vi "VI Anlagengrenzwerte Amium PNS.vi"() -> ()   [LabVIEW 2020, in "Amium PNS.lvlib"]
uses:
  Amium PNS/Amium PNS.lvlib
  Amium PNS/Amium Anlagengrenzwerte PNS.ctl
  Amium PNS/Amium Anlagengrenzwerte-Parameter Anzeige.ctl
  Visualisierungs Elemente/Zahlen-Eingabefeld.ctl
  Visualisierungs Elemente/Button.ctl
  Visualisierungs Elemente/Zahlen-Ausgabefeld.ctl
  Amium PNS/PNS Istwerte_Amium.ctl
  Amium PNS/Amium ErrorCluster.ctl
  Amium PNS/Amium Zustand.ctl
  Amium PNS/SP_Daten.ctl
  Amium PNS/Aktion FGV Amium Daten.ctl
  Seiten/System Einstellungen V2/Aktioen FGV System.ctl
  Amium PNS/AK Kommunikation/Amium Kommandos verwalten Aktionen.ctl
  PNS/Diagnose PNS.vi
  Allgemein/allgemeine Sub-VIs.lvlib
  PNS/PNS.lvlib
  PNS/PNS Anlagenuebersicht einfaerben Aktionen.ctl
  Amium PNS/AK Kommunikation/AK Kommunikation.lvlib
  Seiten/System Einstellungen V2/System Einstellungen V2.lvlib
panel:
  in  "SP":T1
  out "Messgasdruck:":sgl format="%#_5g"
  out "Amium Zustände":T2 items=["Pause", "Aufheizphase", "Standby", "Messen", "Spülen", "Leakcheck"]
  out "Entnahmestelle:":sgl[](array[numeric]) format="%#_5g"
  in  "Port:":u32
  out "Software Version:":string
  out "PNS Istwerte":T3 {"Istwert 14" format="%.1f"; "Istwert 13" format="%.1f"; "Istwert 12" format="%.1f"; "Istwert 11" format="%.1f"; "Istwert 10" format="%.1f"; "Istwert 9" format="%.1f"; "Istwert 8" format="%.1f"; "Istwert 7" format="%.1f"; "Istwert 6" format="%.1f"; "Istwert 5" format="%.1f"; "Istwert 4" format="%.1f"; "Istwert 3" format="%.1f"; "Istwert 2" format="%.1f"; "Istwert 1" format="%.1f"}
  in  "IP-Adresse PNS:":string
  out "Seriennummer:":string
  out "Detail Status:":T4 format="%#_5g"
  out "Status:":T4 format="%#_5g"
  out "Druckluft Störung:":T4 format="%#_5g"
  out "AWC IST:":T4 format="%#_5g"
  out "Error Out":errorcluster caption="Fehlercluster"
  in  "Diag PNS":T5
  in  "Grenzwerte PNS":T6={"Filter:"={"Sollwert"=0.0, "Warn-Min"=0.0, "Warn-Max"=0.0, "Abschalt-Min"=0.0, "Abschalt-Max"=0.0, "Regler"=1}, "Ventilplatte:"={"Sollwert"=0.0, "Warn-Min"=0.0, "Warn-Max"=0.0, "Abschalt-Min"=0.0, "Abschalt-Max"=0.0, "Regler"=1}, "Heizleitung 1:"={"Sollwert"=0.0, "Warn-Min"=0.0, "Warn-Max"=0.0, "Abschalt-Min"=0.0, "Abschalt-Max"=0.0, "Regler"=1}, "Heizleitung 2:"={"Sollwert"=0.0, "Warn-Min"=0.0, "Warn-Max"=0.0, "Abschalt-Min"=0.0, "Abschalt-Max"=0.0, "Regler"=1}, "Heizleitung 3:"={"Sollwert"=0.0, "Warn-Min"=0.0, "Warn-Max"=0.0, "Abschalt-Min"=0.0, "Abschalt-Max"=0.0, "Regler"=1}, "Heizleitung 4:"={"Sollwert"=0.0, "Warn-Min"=0.0, "Warn-Max"=0.0, "Abschalt-Min"=0.0, "Abschalt-Max"=0.0, "Regler"=1}, "Heizleitung 5:"={"Sollwert"=0.0, "Warn-Min"=0.0, "Warn-Max"=0.0, "Abschalt-Min"=0.0, "Abschalt-Max"=0.0, "Regler"=1}, "Heizleitung 6:"={"Sollwert"=0.0, "Warn-Min"=0.0, "Warn-Max"=0.0, "Abschalt-Min"=0.0, "Abschalt-Max"=0.0, "Regler"=1}, "Heizleitung 7:"={"Sollwert"=0.0, "Warn-Min"=0.0, "Warn-Max"=0.0, "Abschalt-Min"=0.0, "Abschalt-Max"=1.0, "Regler"=1}, "Heizleitung 8:"={"Sollwert"=0.0, "Warn-Min"=0.0, "Warn-Max"=0.0, "Abschalt-Min"=0.0, "Abschalt-Max"=0.0, "Regler"=1}, "Heizleitung 9:"={"Sollwert"=0.0, "Warn-Min"=0.0, "Warn-Max"=0.0, "Abschalt-Min"=0.0, "Abschalt-Max"=0.0, "Regler"=1}, "Heizleitung 10:"={"Sollwert"=0.0, "Warn-Min"=0.0, "Warn-Max"=0.0, "Abschalt-Min"=0.0, "Abschalt-Max"=0.0, "Regler"=1}, "Heizleitung 11:"={"Sollwert"=0.0, "Warn-Min"=0.0, "Warn-Max"=0.0, "Abschalt-Min"=0.0, "Abschalt-Max"=0.0, "Regler"=1}, "Heizleitung 12:"={"Sollwert"=0.0, "Warn-Min"=0.0, "Warn-Max"=0.0, "Abschalt-Min"=0.0, "Abschalt-Max"=0.0, "Regler"=1}} {"Heizleitung 12:"."Regler" items=["aktiv", "inaktiv"]; "Heizleitung 12:"."Abschalt-Max" format="%#_5g"; "Heizleitung 12:"."Abschalt-Min" format="%#_5g"; "Heizleitung 12:"."Warn-Max" format="%#_5g"; "Heizleitung 12:"."Warn-Min" format="%#_5g"; "Heizleitung 12:"."Sollwert" format="%#_5g"; "Heizleitung 11:"."Regler" items=["aktiv", "inaktiv"]; "Heizleitung 11:"."Abschalt-Max" format="%#_5g"; "Heizleitung 11:"."Abschalt-Min" format="%#_5g"; "Heizleitung 11:"."Warn-Max" format="%#_5g"; "Heizleitung 11:"."Warn-Min" format="%#_5g"; "Heizleitung 11:"."Sollwert" format="%#_5g"; "Heizleitung 10:"."Regler" items=["aktiv", "inaktiv"]; "Heizleitung 10:"."Abschalt-Max" format="%#_5g"; "Heizleitung 10:"."Abschalt-Min" format="%#_5g"; "Heizleitung 10:"."Warn-Max" format="%#_5g"; "Heizleitung 10:"."Warn-Min" format="%#_5g"; "Heizleitung 10:"."Sollwert" format="%#_5g"; "Heizleitung 9:"."Regler" items=["aktiv", "inaktiv"]; "Heizleitung 9:"."Abschalt-Max" format="%#_5g"; "Heizleitung 9:"."Abschalt-Min" format="%#_5g"; "Heizleitung 9:"."Warn-Max" format="%#_5g"; "Heizleitung 9:"."Warn-Min" format="%#_5g"; "Heizleitung 9:"."Sollwert" format="%#_5g"; "Heizleitung 8:"."Regler" items=["aktiv", "inaktiv"]; "Heizleitung 8:"."Abschalt-Max" format="%#_5g"; "Heizleitung 8:"."Abschalt-Min" format="%#_5g"; "Heizleitung 8:"."Warn-Max" format="%#_5g"; "Heizleitung 8:"."Warn-Min" format="%#_5g"; "Heizleitung 8:"."Sollwert" format="%#_5g"; "Heizleitung 7:"."Regler" items=["aktiv", "inaktiv"]; "Heizleitung 7:"."Abschalt-Max" format="%#_5g"; "Heizleitung 7:"."Abschalt-Min" format="%#_5g"; "Heizleitung 7:"."Warn-Max" format="%#_5g"; "Heizleitung 7:"."Warn-Min" format="%#_5g"; "Heizleitung 7:"."Sollwert" format="%#_5g"; "Heizleitung 6:"."Regler" items=["aktiv", "inaktiv"]; "Heizleitung 6:"."Abschalt-Max" format="%#_5g"; "Heizleitung 6:"."Abschalt-Min" format="%#_5g"; "Heizleitung 6:"."Warn-Max" format="%#_5g"; "Heizleitung 6:"."Warn-Min" format="%#_5g"; "Heizleitung 6:"."Sollwert" format="%#_5g"; "Heizleitung 5:"."Regler" items=["aktiv", "inaktiv"]; "Heizleitung 5:"."Abschalt-Max" format="%#_5g"; "Heizleitung 5:"."Abschalt-Min" format="%#_5g"; "Heizleitung 5:"."Warn-Max" format="%#_5g"; "Heizleitung 5:"."Warn-Min" format="%#_5g"; "Heizleitung 5:"."Sollwert" format="%#_5g"; "Heizleitung 4:"."Regler" items=["aktiv", "inaktiv"]; "Heizleitung 4:"."Abschalt-Max" format="%#_5g"; "Heizleitung 4:"."Abschalt-Min" format="%#_5g"; "Heizleitung 4:"."Warn-Max" format="%#_5g"; "Heizleitung 4:"."Warn-Min" format="%#_5g"; "Heizleitung 4:"."Sollwert" format="%#_5g"; "Heizleitung 3:"."Regler" items=["aktiv", "inaktiv"]; "Heizleitung 3:"."Abschalt-Max" format="%#_5g"; "Heizleitung 3:"."Abschalt-Min" format="%#_5g"; "Heizleitung 3:"."Warn-Max" format="%#_5g"; "Heizleitung 3:"."Warn-Min" format="%#_5g"; "Heizleitung 3:"."Sollwert" format="%#_5g"; "Heizleitung 2:"."Regler" items=["aktiv", "inaktiv"]; "Heizleitung 2:"."Abschalt-Max" format="%#_5g"; "Heizleitung 2:"."Abschalt-Min" format="%#_5g"; "Heizleitung 2:"."Warn-Max" format="%#_5g"; "Heizleitung 2:"."Warn-Min" format="%#_5g"; "Heizleitung 2:"."Sollwert" format="%#_5g"; "Heizleitung 1:"."Regler" items=["aktiv", "inaktiv"]; "Heizleitung 1:"."Abschalt-Max" format="%#_5g"; "Heizleitung 1:"."Abschalt-Min" format="%#_5g"; "Heizleitung 1:"."Warn-Max" format="%#_5g"; "Heizleitung 1:"."Warn-Min" format="%#_5g"; "Heizleitung 1:"."Sollwert" format="%#_5g"; "Ventilplatte:"."Regler" items=["aktiv", "inaktiv"]; "Ventilplatte:"."Abschalt-Max" format="%#_5g"; "Ventilplatte:"."Abschalt-Min" format="%#_5g"; "Ventilplatte:"."Warn-Max" format="%#_5g"; "Ventilplatte:"."Warn-Min" format="%#_5g"; "Ventilplatte:"."Sollwert" format="%#_5g"; "Filter:"."Regler" items=["aktiv", "inaktiv"]; "Filter:"."Abschalt-Max" format="%#_5g"; "Filter:"."Abschalt-Min" format="%#_5g"; "Filter:"."Warn-Max" format="%#_5g"; "Filter:"."Warn-Min" format="%#_5g"; "Filter:"."Sollwert" format="%#_5g"}
  out "Fehler Cluster":T9
  # "Amium Anlagengrenzwerte PNS"
  # "Allgemeine Werte"
  # "Abschaltgrenzen"
  # "Warngrenzen"
  # "Regelung \naktiv/inaktiv"
  # "Parameter"
  # "Istwert"
  # "Sollwert"
  # "Min"
  # "Max"
  # "Min"
  # "Max"
  # "Heizleitung 1:"
  # "Diagnosewerte"
  # "Heizleitung 2:"
  # "Heizleitung 3:"
  # "Heizleitung 4:"
  # "Heizleitung 5:"
  # "Heizleitung 6:"
  # "Heizleitung 7:"
  # "Heizleitung 8:"
  # "Heizleitung 9:"
  # "Heizleitung 10:"
  # "Ofen / Filter:"
  # "HL Zuleitung:"
  # "Wanddurchführung:"
  # "AddOn:"
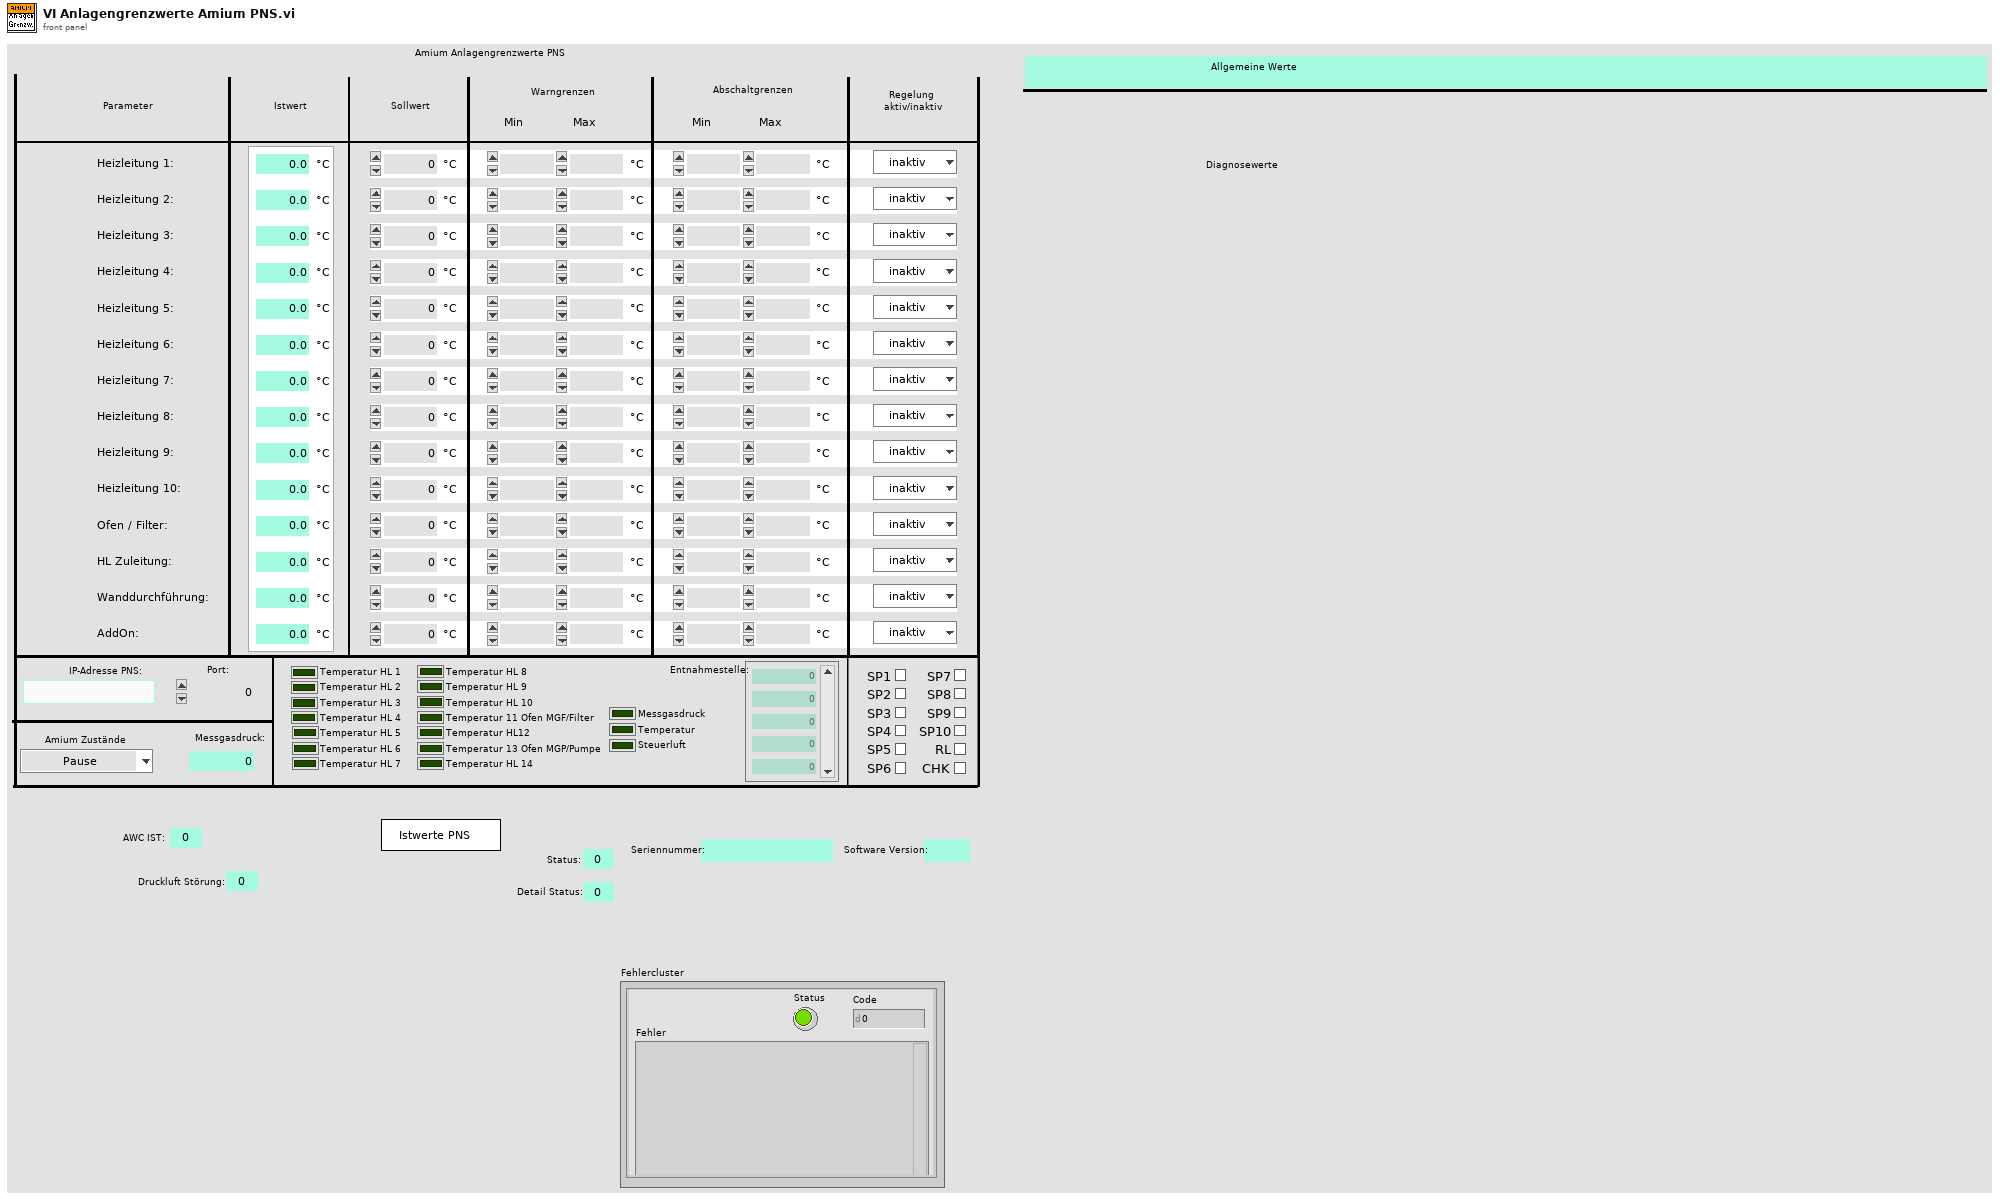
[diagram p1: front panel]
types:
  T1 = typedef "Amium PNS.lvlib/SP_Daten.ctl" = cluster{"SP1":bool, "SP2":bool, "SP3":bool, "SP4":bool, "SP5":bool, "SP6":bool, "SP7":bool, "SP8":bool, "SP9":bool, "SP10":bool, "RL":bool, "CHK":bool}
  T2 = typedef "Amium PNS.lvlib/Amium Zustand.ctl" = u16
  T3 = typedef "Amium PNS.lvlib/PNS Istwerte_Amium.ctl" = cluster{"Istwert 1":sgl, "Istwert 2":sgl, "Istwert 3":sgl, "Istwert 4":sgl, "Istwert 5":sgl, "Istwert 6":sgl, "Istwert 7":sgl, "Istwert 8":sgl, "Istwert 9":sgl, "Istwert 10":sgl, "Istwert 11":sgl, "Istwert 12":sgl, "Istwert 13":sgl, "Istwert 14":sgl}
  T4 = typedef "Zahlen-Ausgabefeld.ctl" = sgl
  T5 = typedef "Button.ctl" = bool
  T6 = typedef "Amium PNS.lvlib/Amium Anlagengrenzwerte PNS.ctl" = cluster{"Filter:":T7, "Ventilplatte:":T7, "Heizleitung 1:":T7, "Heizleitung 2:":T7, "Heizleitung 3:":T7, "Heizleitung 4:":T7, "Heizleitung 5:":T7, "Heizleitung 6:":T7, "Heizleitung 7:":T7, "Heizleitung 8:":T7, "Heizleitung 9:":T7, "Heizleitung 10:":T7, "Heizleitung 11:":T7, "Heizleitung 12:":T7}
  T7 = typedef "Amium PNS.lvlib/Amium Anlagengrenzwerte-Parameter Anzeige.ctl" = cluster{"Sollwert":T8, "Warn-Min":T8, "Warn-Max":T8, "Abschalt-Min":T8, "Abschalt-Max":T8, "Regler":u16}
  T8 = typedef "Zahlen-Eingabefeld.ctl" = sgl
  T9 = typedef "Amium PNS.lvlib/Amium ErrorCluster.ctl" = cluster{"Messgasdruck":bool, "Temperatur":bool, "Steuerluft":bool, "Temperatur HL 1":bool, "Temperatur HL 2":bool, "Temperatur HL 3":bool, "Temperatur HL 4":bool, "Temperatur HL 5":bool, "Temperatur HL 6":bool, "Temperatur HL 7":bool, "Temperatur HL 8":bool, "Temperatur HL 9":bool, "Temperatur HL 10":bool, "Temperatur 11 Ofen MGF/Filter":bool, "Temperatur HL12":bool, "Temperatur 13 Ofen MGP/Pumpe":bool, "Temperatur HL 14":bool}
  T10 = enum8{"Enabled", "Disabled", "Disabled and Grayed Out"}
  T11 = typedef "System Einstellungen V2.lvlib/Aktioen FGV System.ctl" = enum16{"lesen", "laden", "speichern", "Optionen schreiben", "Zeitstempel", "Reset BMP", "Reset SQP", "Wartung", "Werkseinstellung"}
  T12 = typedef "Amium PNS.lvlib/Aktion FGV Amium Daten.ctl" = enum16{"lesen", "Komm Daten", "Daten", "Error", "Regler", "Grenzwerte", "laden", "speichern"}
  T13 = typedef "PNS.lvlib/PNS Anlagenuebersicht einfaerben Aktionen.ctl" = enum16{"lesen", "prüfen", "initialisieren"}
  T14 = typedef "System Einstellungen V2.lvlib/Optionen.ctl" = cluster{"Störmeldep.":bool, "Betriebszustände":bool, "LN2 Befüllung":bool, "Klimaanlage ?":bool, "AK in ppm":bool, "log Cal-Gas":bool, "log 0-Gas":bool, "log CG zu PNS":bool, "Reserve":bool, "Durchflusssensor 0-5V":bool, "PNS?":bool, "Container":bool, "Mit N2 spülen":bool, "Span Gas Auswahl":T15, "VFS 1":bool, "VFS 2":bool, "VFS 3":bool, "VFS 4":bool, "TRE08":bool, "Leakcheck vor Kal":bool, "Amium 10-Fach":bool, "Verticale Scrollbar aktiv":bool, "Loggingtakt":bool, "SP laden speichern":u16}
  T15 = typedef "Funktionstasten.lvlib/Spaneingang.ctl" = u16
  T16 = typedef "Amium PNS.lvlib/Kommunikation Daten Cluster.ctl" = cluster{"IP Adresse":string, "Port":i16}
  T17 = typedef "Amium PNS.lvlib/AK Kommunikation.lvlib/Amium Kommandos verwalten Aktionen.ctl" = enum16{"lesen", "setzen Ende", "setzen Pos1", "senden", "initalisieren", "prüfen", "Kommandos"}
  T18 = cluster{"Filter:":cluster{"Sollwert":bool, "Warn-Min":bool, "Warn-Max":bool, "Abschalt-Min":bool, "Abschalt-Max":bool, "Regler":bool}, "Ventilplatte:":cluster{"Sollwert":bool, "Warn-Min":bool, "Warn-Max":bool, "Abschalt-Min":bool, "Abschalt-Max":bool, "Regler":bool}, "Heizleitung 1:":cluster{"Sollwert":bool, "Warn-Min":bool, "Warn-Max":bool, "Abschalt-Min":bool, "Abschalt-Max":bool, "Regler":bool}, "Heizleitung 2:":cluster{"Sollwert":bool, "Warn-Min":bool, "Warn-Max":bool, "Abschalt-Min":bool, "Abschalt-Max":bool, "Regler":bool}, "Heizleitung 3:":cluster{"Sollwert":bool, "Warn-Min":bool, "Warn-Max":bool, "Abschalt-Min":bool, "Abschalt-Max":bool, "Regler":bool}, "Heizleitung 4:":cluster{"Sollwert":bool, "Warn-Min":bool, "Warn-Max":bool, "Abschalt-Min":bool, "Abschalt-Max":bool, "Regler":bool}, "Heizleitung 5:":cluster{"Sollwert":bool, "Warn-Min":bool, "Warn-Max":bool, "Abschalt-Min":bool, "Abschalt-Max":bool, "Regler":bool}, "Heizleitung 6:":cluster{"Sollwert":bool, "Warn-Min":bool, "Warn-Max":bool, "Abschalt-Min":bool, "Abschalt-Max":bool, "Regler":bool}, "Heizleitung 7:":cluster{"Sollwert":bool, "Warn-Min":bool, "Warn-Max":bool, "Abschalt-Min":bool, "Abschalt-Max":bool, "Regler":bool}, "Heizleitung 8:":cluster{"Sollwert":bool, "Warn-Min":bool, "Warn-Max":bool, "Abschalt-Min":bool, "Abschalt-Max":bool, "Regler":bool}, "Heizleitung 9:":cluster{"Sollwert":bool, "Warn-Min":bool, "Warn-Max":bool, "Abschalt-Min":bool, "Abschalt-Max":bool, "Regler":bool}, "Heizleitung 10:":cluster{"Sollwert":bool, "Warn-Min":bool, "Warn-Max":bool, "Abschalt-Min":bool, "Abschalt-Max":bool, "Regler":bool}, "Heizleitung 11:":cluster{"Sollwert":bool, "Warn-Min":bool, "Warn-Max":bool, "Abschalt-Min":bool, "Abschalt-Max":bool, "Regler":bool}, "Heizleitung 12:":cluster{"Sollwert":bool, "Warn-Min":bool, "Warn-Max":bool, "Abschalt-Min":bool, "Abschalt-Max":bool, "Regler":bool}}
  T19 = cluster{"Sollwert":bool, "Warn-Min":bool, "Warn-Max":bool, "Abschalt-Min":bool, "Abschalt-Max":bool, "Regler":bool}[]
  T20 = typedef "Amium PNS.lvlib/Daten Cluster.ctl" = cluster{"Amium Zustände":T2, "Samplepoint am PNS":i16, "Gerätekennung":string, "aktiver Samplepoint":i16[], "Messgasdruck":sgl}
  T21 = typedef "Amium PNS.lvlib/Temperaturregler Cluster.ctl" = cluster{"Istwert":sgl, "Sollwert":sgl, "Stellgröße":sgl, "Status":sgl, "Error":sgl}
  T22 = cluster{"Istwert":sgl, "Istwert":sgl, "Istwert":sgl, "Istwert":sgl, "Istwert":sgl, "Istwert":sgl, "Istwert":sgl, "Istwert":sgl, "Istwert":sgl, "Istwert":sgl, "Istwert":sgl, "Istwert":sgl, "Istwert":sgl, "Istwert":sgl}
  T23 = cluster{"[0]":T7, "[1]":T7, "[2]":T7, "[3]":T7, "[4]":T7, "[5]":T7, "[6]":T7, "[7]":T7, "[8]":T7, "[9]":T7, "[10]":T7, "[11]":T7, "[12]":T7, "[13]":T7}
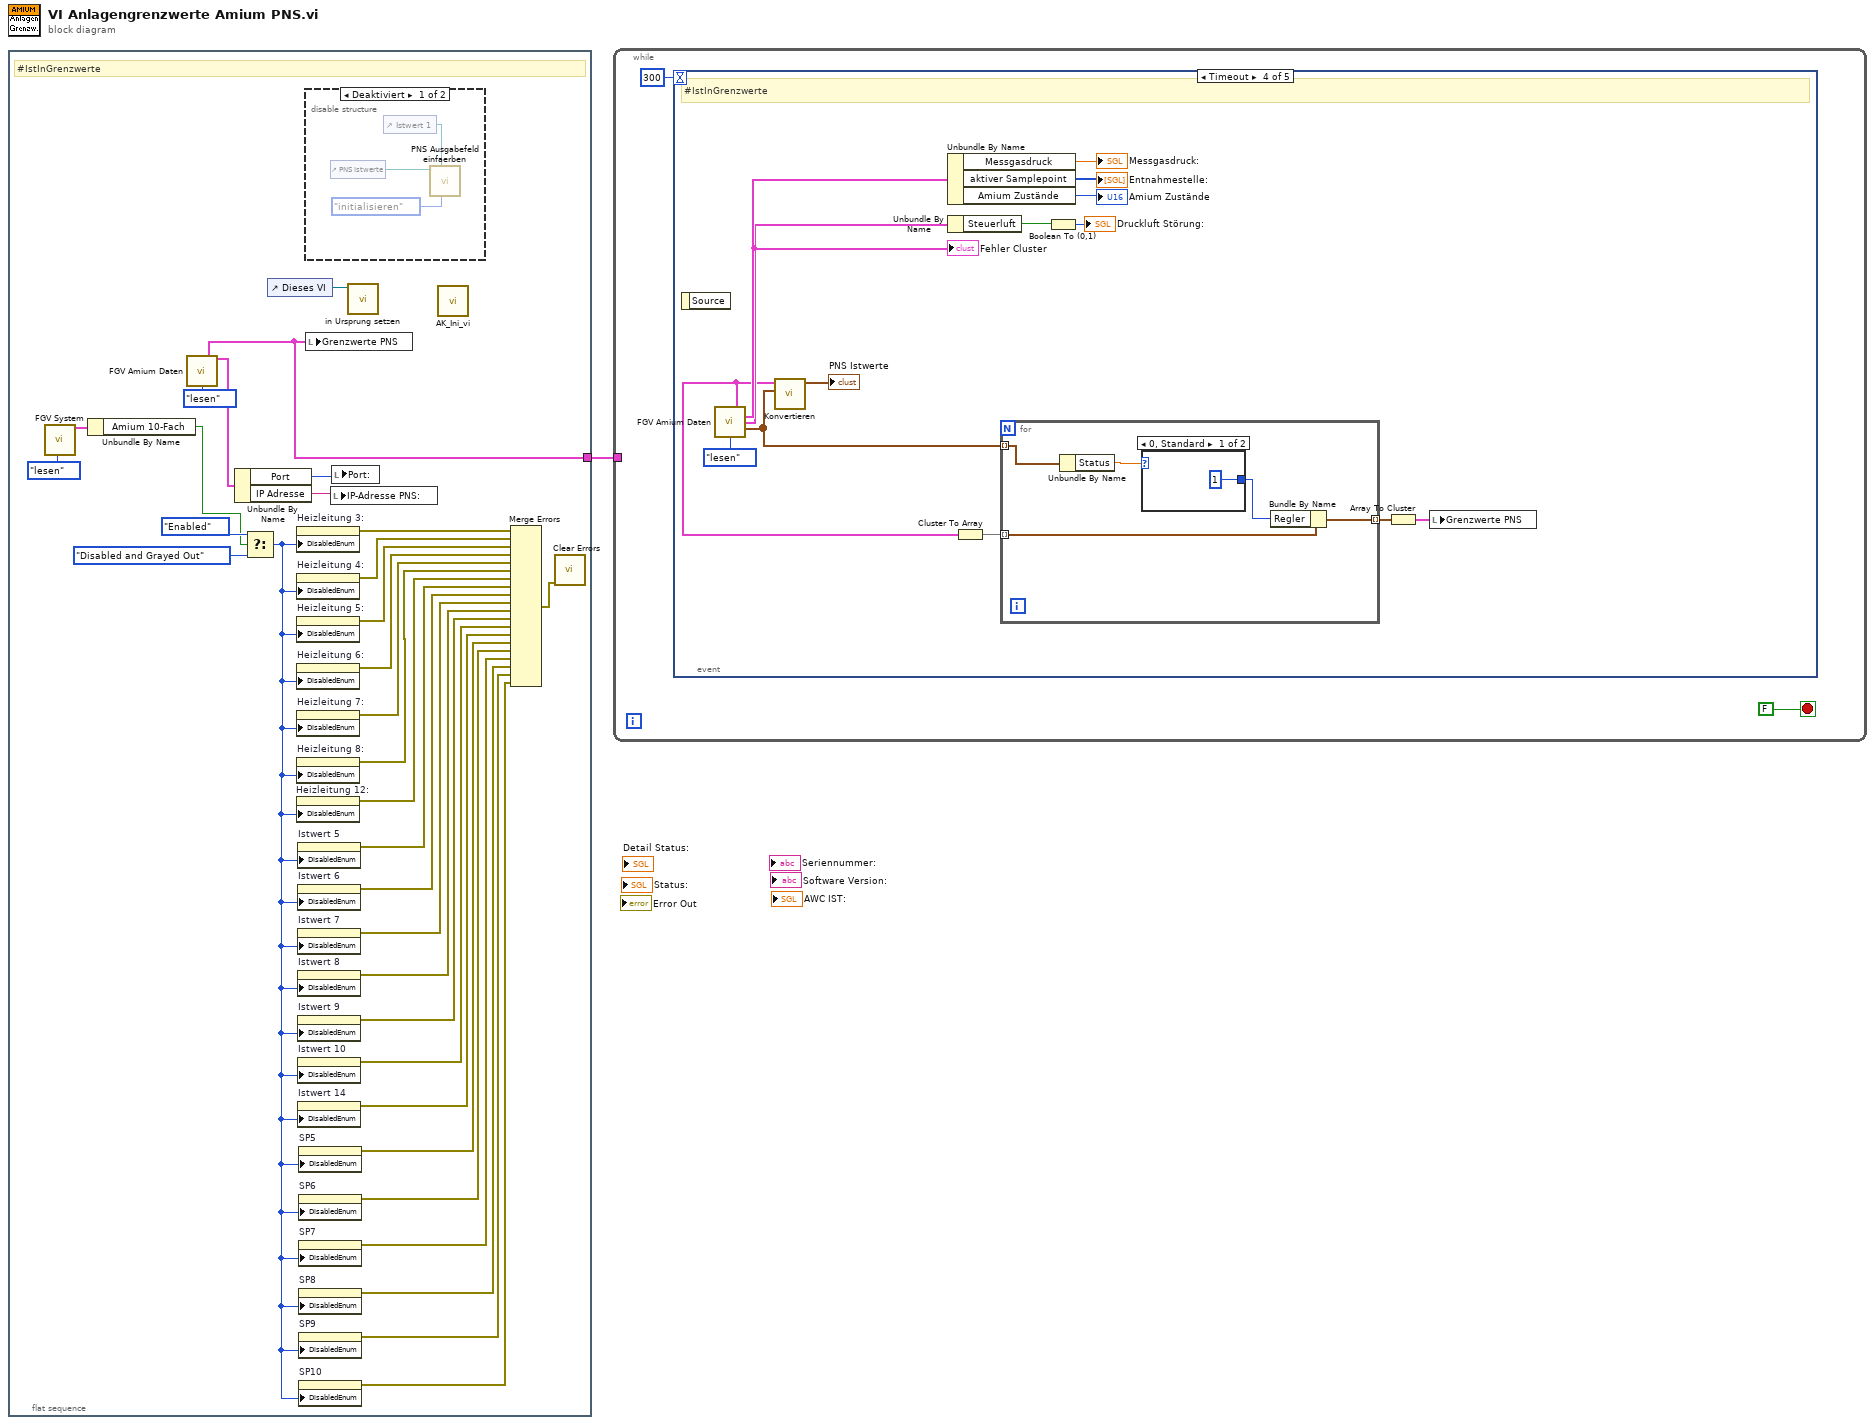
[diagram p0: block diagram]
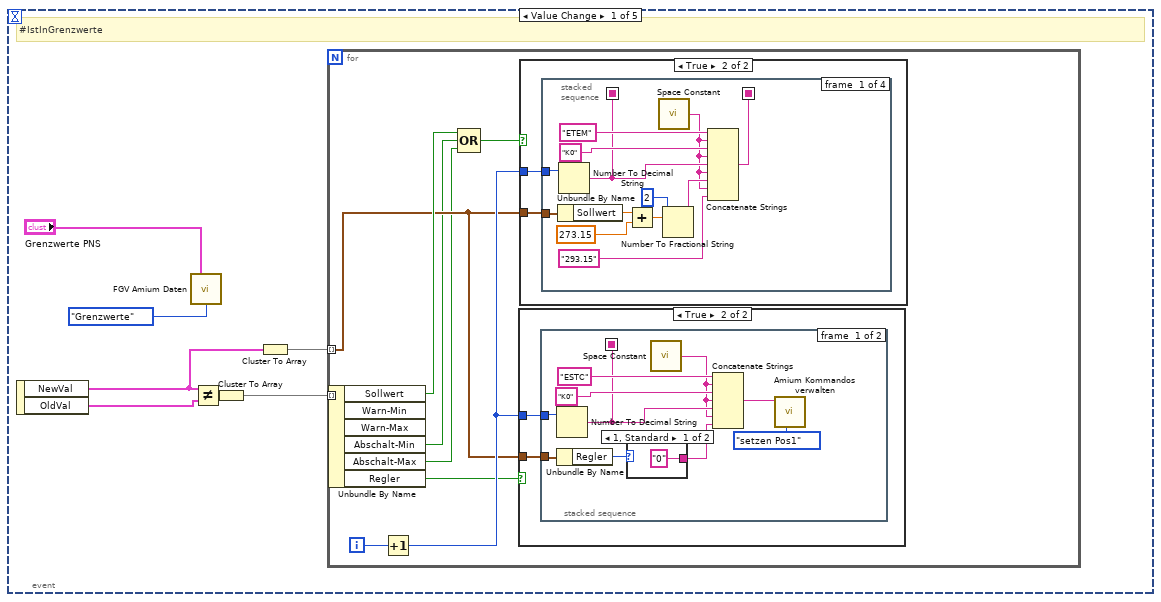
[diagram p3: hidden frame]
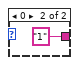
[diagram p5: hidden frame]
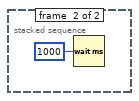
[diagram p6: hidden frame]
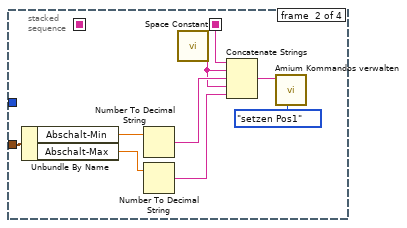
[diagram p8: hidden frame]
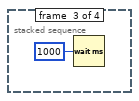
[diagram p9: hidden frame]
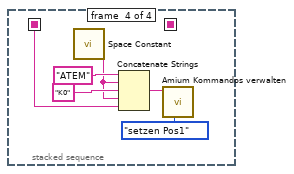
[diagram p10: hidden frame]
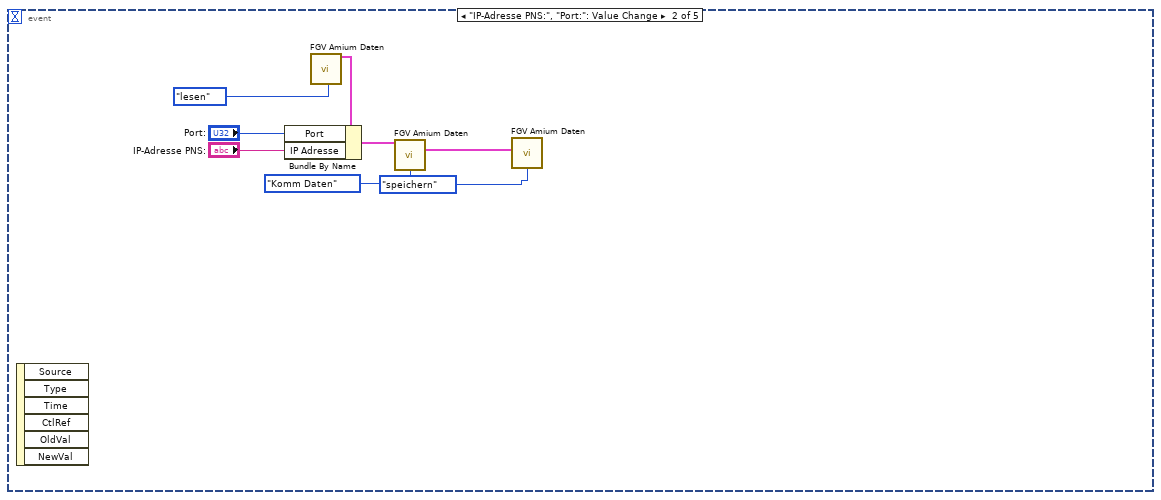
[diagram p11: hidden frame]
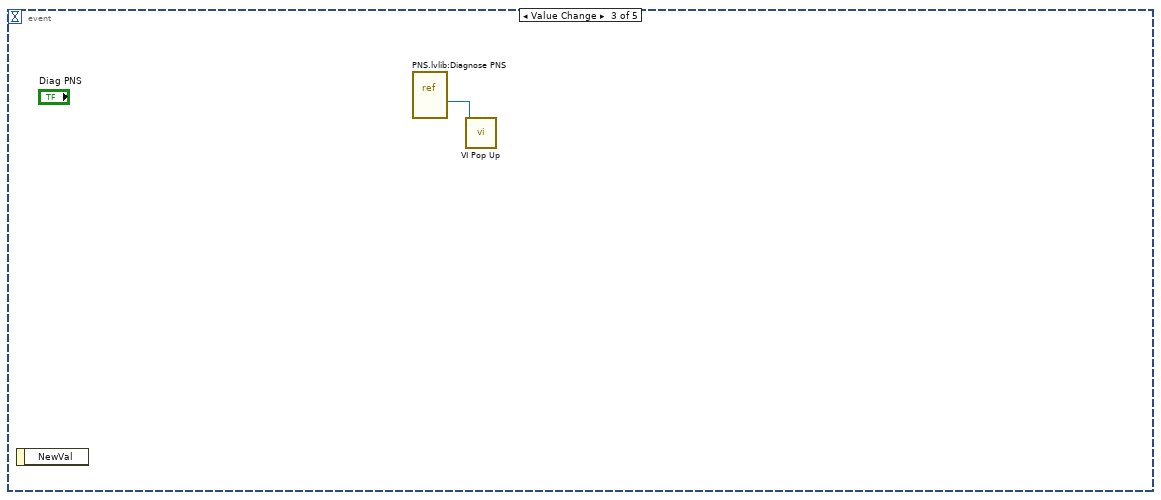
[diagram p12: hidden frame]
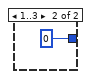
[diagram p13: hidden frame]
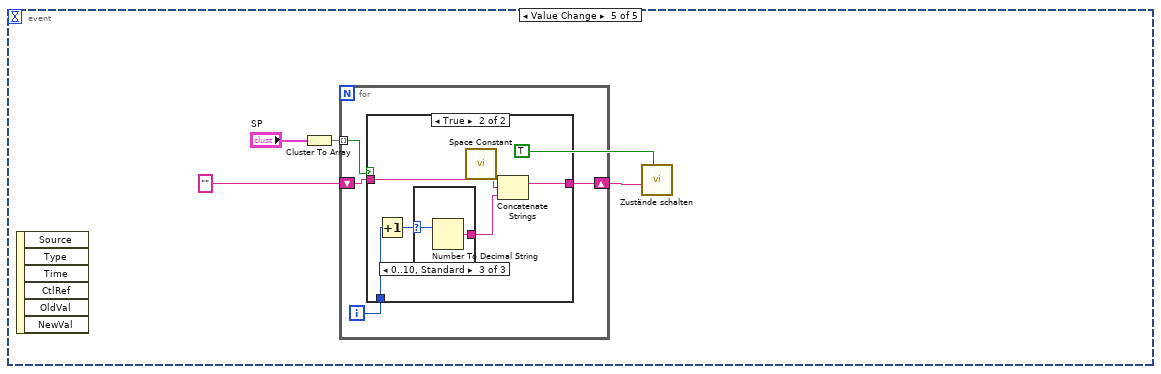
[diagram p14: hidden frame]
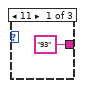
[diagram p16: hidden frame]
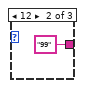
[diagram p17: hidden frame]
diagram:
  n1 = flat-sequence {
    tunnel: [w32] -> w1
    frame #0 {
      # "#IstInGrenzwerte"
      n2 = call "FGV System.vi"("Aktionen"=Aktioen_FGV_System."lesen") -> ("Optionen"=w27:T14)  [unwired: 12 in, 6 out]
      n3 = Unbundle By Name(w27) -> ("Amium 10-Fach"=w2:bool)
      n4 = call "FGV Amium Daten.vi"("Aktion"=Aktion_FGV_Amium_Daten."lesen") -> ("Grenzwerte PNS"=w32:T6, "Amium Komm Daten"=w31:T16)  [unwired: 9 in, 4 out]
      n5 = Unbundle By Name(w31) -> ("Port"=w30:i16, "IP Adresse"=w29:string)
      n6 = Select(t=T10."Enabled", s=w2, f=T10."Disabled and Grayed Out" ("Deaktiviert")) -> (s? t:f=w6:T10)
      n7 = control-ref of="Dieses VI"() -> (w34:refnum<vi>)
      n8 = property on="Heizleitung 3:" class="Cluster (strikt)"("DisabledEnum"=w6) -> (error out=w24:errorcluster)  [unwired: 2 in, 1 out]
      n9 = property on="Heizleitung 4:" class="Cluster (strikt)"("DisabledEnum"=w6) -> (error out=w23:errorcluster)  [unwired: 2 in, 1 out]
      n10 = property on="Heizleitung 5:" class="Cluster (strikt)"("DisabledEnum"=w6) -> (error out=w22:errorcluster)  [unwired: 2 in, 1 out]
      n11 = property on="Heizleitung 6:" class="Cluster (strikt)"("DisabledEnum"=w6) -> (error out=w21:errorcluster)  [unwired: 2 in, 1 out]
      n12 = property on="Heizleitung 7:" class="Cluster (strikt)"("DisabledEnum"=w6) -> (error out=w20:errorcluster)  [unwired: 2 in, 1 out]
      n13 = property on="Heizleitung 8:" class="Cluster (strikt)"("DisabledEnum"=w6) -> (error out=w19:errorcluster)  [unwired: 2 in, 1 out]
      n14 = property on="Heizleitung 12:" class="Cluster (strikt)"("DisabledEnum"=w6) -> (error out=w18:errorcluster)  [unwired: 2 in, 1 out]
      n15 = property on="Istwert 5" class="DigWert (strikt)"("DisabledEnum"=w6) -> (error out=w16:errorcluster)  [unwired: 2 in, 1 out]
      n16 = property on="Istwert 6" class="DigWert (strikt)"("DisabledEnum"=w6) -> (error out=w15:errorcluster)  [unwired: 2 in, 1 out]
      n17 = property on="Istwert 7" class="DigWert (strikt)"("DisabledEnum"=w6) -> (error out=w14:errorcluster)  [unwired: 2 in, 1 out]
      n18 = property on="Istwert 8" class="DigWert (strikt)"("DisabledEnum"=w6) -> (error out=w13:errorcluster)  [unwired: 2 in, 1 out]
      n19 = property on="Istwert 9" class="DigWert (strikt)"("DisabledEnum"=w6) -> (error out=w12:errorcluster)  [unwired: 2 in, 1 out]
      n20 = property on="Istwert 10" class="DigWert (strikt)"("DisabledEnum"=w6) -> (error out=w11:errorcluster)  [unwired: 2 in, 1 out]
      n21 = property on="Istwert 14" class="DigWert (strikt)"("DisabledEnum"=w6) -> (error out=w10:errorcluster)  [unwired: 2 in, 1 out]
      n22 = property on="SP5" class="Bool. (strikt)"("DisabledEnum"=w6) -> (error out=w9:errorcluster)  [unwired: 2 in, 1 out]
      n23 = property on="SP6" class="Bool. (strikt)"("DisabledEnum"=w6) -> (error out=w8:errorcluster)  [unwired: 2 in, 1 out]
      n24 = property on="SP7" class="Bool. (strikt)"("DisabledEnum"=w6) -> (error out=w7:errorcluster)  [unwired: 2 in, 1 out]
      n25 = property on="SP8" class="Bool. (strikt)"("DisabledEnum"=w6) -> (error out=w5:errorcluster)  [unwired: 2 in, 1 out]
      n26 = property on="SP9" class="Bool. (strikt)"("DisabledEnum"=w6) -> (error out=w4:errorcluster)  [unwired: 2 in, 1 out]
      n27 = property on="SP10" class="Bool. (strikt)"("DisabledEnum"=w6) -> (error out=w3:errorcluster)  [unwired: 2 in, 1 out]
      n28 = disable-structure shown="Deaktiviert" {
        frame Disabled {
          n29 = control-ref of="PNS Istwerte"() -> (w36:refnum<vi>)
          n30 = control-ref of="Istwert 1"() -> (w35:refnum<vi>)
          n31 = call "PNS Ausgabefeld einfaerben.vi"("Aktionen"=PNS_Anlagenuebersicht_einfaerben_Aktionen."initialisieren", "FeldTyp (Eingang)"=w35, "PNS Istwerte"=w36) -> ()  [unwired: 9 in]
        }
        frame Enabled {
        }
      }
      n32 = local write "Grenzwerte PNS"(w32) -> ()
      n33 = local write "IP-Adresse PNS:"(w29) -> ()
      n34 = local write "Port:"(w30) -> ()
      n35 = call "in Ursprung setzen.vi"("VI Referenz"=w34) -> ()  [unwired: 11 in]
      n36 = call "AK_Ini_vi.vi"() -> ()  [unwired: 12 in]
      n37 = Merge Errors(w24, w23, w22, w21, w20, w19, w18, w16, w15, w14, w13, w12, w11, w10, w9, w8, w7, w5, w4, w3) -> (w17:errorcluster)
      n38 = call <vilib>:"Clear Errors.vi"("error in (no error)"=w17) -> ()  [unwired: 5 in, 2 out]
    }
  }
  n39 = while {
    tunnel: w1 -> [_]
    stop <- FALSE stop-if-true
    n40 = event shown="[3] Timeout" {
      selector: _ -> [_ _ _ _ _]
      dyn-events: _ -> [_ _ _ _ _]
      timeout: 300 -> [_ _ _ _ _]
      event Value Change {
        # "#IstInGrenzwerte"
        n41 = event-data() -> ("NewVal"=w41:T6, "OldVal"=w44:T6)  [unwired: 1 out]
        n42 = call "FGV Amium Daten.vi"("Grenzwerte PNS"="Grenzwerte PNS", "Aktion"=Aktion_FGV_Amium_Daten."Grenzwerte") -> ()  [unwired: 8 in, 6 out]
        n43 = Not Equal?(x=w41, y=w44) -> (x != y?=w43:T18)
        n44 = Cluster To Array(cluster=w43) -> (array=w42:T19)
        n45 = Cluster To Array(cluster=w41) -> (array=w40:T7[])
        n46 = for {
          tunnel: w42 -> [w55] mode=indexing
          tunnel: w40 -> [w51] mode=indexing
          i -> [w53]
          n47 = Unbundle By Name(w55) -> ("Sollwert"=w54:bool, "Abschalt-Min"=w48:bool, "Abschalt-Max"=w47:bool, "Regler"=w50:bool)  [unwired: 2 out]
          n48 = Increment(x=w53) -> (x+1=w52:i32)
          n49 = Compound Arithmetic op=OR ("Mehrfacharithmetik")(w54, w48, w47) -> (w49:bool)
          n50 = case shown="True" w50 {
            tunnel: w52 -> [_ w57]
            tunnel: w51 -> [_ w56]
            frame False {
            }
            frame True {
              n51 = stacked-sequence {
                seq-local: [w63 _] -> [_ _]
                tunnel: w57 -> [w64 _]
                tunnel: w56 -> [w62 _]
                frame #0 {
                  n52 = Number To Decimal String(number=w64) -> (decimal integer string=w63:string)  [unwired: 1 in]
                  n53 = Unbundle By Name(w62) -> ("Regler"=w61:u16)
                  n54 = case shown="1, Standard" w61 {
                    tunnel: ["0" "1"] -> w60
                    frame 1, Default {
                    }
                    frame 0 {
                    }
                  }
                  n55 = call <vilib>:"Space Constant.vi"() -> ("String"=w59:string)
                  n56 = Concatenate Strings("ESTC", w59, "K0" ("Element"), w59, w63, w59, w60) -> (w58:string)
                  n57 = call "Amium Kommandos verwalten.vi"("Aktionen"=Amium_Kommandos_verwalten_Aktionen."setzen Pos1", "neues Kommando"=w58) -> ()  [unwired: 7 in, 3 out]
                }
                frame #1 {
                  n58 = Wait (ms)(milliseconds to wait=u32 1000 ("Zu wartende ms")) -> ()  [unwired: 1 out]
                }
              }
            }
          }
          n59 = case shown="True" w49 {
            tunnel: w52 -> [_ w72]
            tunnel: w51 -> [_ w71]
            frame False {
            }
            frame True {
              n60 = stacked-sequence {
                seq-local: [w76 _ _ _] -> [_ _ _ w98]
                seq-local: [w75 _ _ _] -> [_ w88 _ _]
                tunnel: w72 -> [w83 _ _ _]
                tunnel: w71 -> [w82 w93 _ _]
                frame #0 {
                  n61 = Unbundle By Name(w82) -> ("Sollwert"=w80:T8)
                  n62 = Number To Decimal String(number=w83) -> (decimal integer string=w76:string)  [unwired: 1 in]
                  n63 = Add(x=w80, y=273.15) -> (x+y=w78:dbl)
                  n64 = call <vilib>:"Space Constant.vi"() -> ("String"=w74:string)
                  n65 = Number To Fractional String(number=w78, precision (6)=i16 2 ("Breite (-)")) -> (F-format string=w79:string)  [unwired: 2 in]
                  n66 = Concatenate Strings("ETEM", w74, "K0" ("Element"), w74, w76, w74, w79, w74, "293.15" ("String")) -> (w75:string)
                }
                frame #1 {
                  n67 = Unbundle By Name(w93) -> ("Abschalt-Min"=w87:T8, "Abschalt-Max"=w86:T8)
                  n68 = Number To Decimal String(number=w87) -> (decimal integer string=w92:string)  [unwired: 1 in]
                  n69 = Number To Decimal String(number=w86) -> (decimal integer string=w91:string)  [unwired: 1 in]
                  n70 = call <vilib>:"Space Constant.vi"() -> ("String"=w89:string)
                  n71 = Concatenate Strings(w88, w89, w92, w89, w91) -> (w90:string)
                  n72 = call "Amium Kommandos verwalten.vi"("Aktionen"=Amium_Kommandos_verwalten_Aktionen."setzen Pos1", "neues Kommando"=w90) -> ()  [unwired: 7 in, 3 out]
                }
                frame #2 {
                  n73 = Wait (ms)(milliseconds to wait=u32 1000 ("Zu wartende ms")) -> ()  [unwired: 1 out]
                }
                frame #3 {
                  n74 = call <vilib>:"Space Constant.vi"() -> ("String"=w96:string)
                  n75 = Concatenate Strings("ATEM", w96, "K0", w96, w98) -> (w97:string)
                  n76 = call "Amium Kommandos verwalten.vi"("Aktionen"=Amium_Kommandos_verwalten_Aktionen."setzen Pos1", "neues Kommando"=w97) -> ()  [unwired: 7 in, 3 out]
                }
              }
            }
          }
        }
      }
      event "IP-Adresse PNS:", "Port:": Value Change {
        n77 = event-data() -> ()  [unwired: 7 out]
        n78 = call "FGV Amium Daten.vi"("Aktion"=Aktion_FGV_Amium_Daten."lesen") -> ("Amium Komm Daten"=w107:T16)  [unwired: 9 in, 5 out]
        n79 = Bundle By Name(cluster=w107, "Port"="Port:", "IP Adresse"="IP-Adresse PNS:") -> (w105:T16)
        n80 = call "FGV Amium Daten.vi"("Amium Komm  Daten"=w105, "Aktion"=Aktion_FGV_Amium_Daten."Komm Daten") -> ("Amium Daten"=w102:T20)  [unwired: 8 in, 5 out]
        n81 = call "FGV Amium Daten.vi"("Amium Daten"=w102, "Aktion"=Aktion_FGV_Amium_Daten."speichern") -> ()  [unwired: 8 in, 6 out]
      }
      event Value Change {
        n82 = event-data() -> ()  [unwired: 2 out]
        n83 = vi-ref "PNS.lvlib:Diagnose PNS.vi"() -> (w110:refnum<vi>)
        n84 = call "VI Pop Up.vi"("VI Referenz"=w110) -> ()  [unwired: 11 in]
      }
      event Timeout {
        # "#IstInGrenzwerte"
        n85 = event-data() -> ()  [unwired: 2 out]
        n86 = call "FGV Amium Daten.vi"("Aktion"=Aktion_FGV_Amium_Daten."lesen") -> ("Grenzwerte PNS"=w114:T6, "Amium Daten"=w122:T20, "Fehler Cluster"=w121:T9, "Regler"=w115:T21[])  [unwired: 9 in, 2 out]
        "Fehler Cluster" <- w121
        n87 = call "Konvertieren.vi"("Regler"=w115, "Grenzwerte PNS (Eingang)"=w114) -> ("Cluster"=→"PNS Istwerte":T22)  [unwired: 8 in, 1 out]
        n88 = Unbundle By Name(w122) -> ("Messgasdruck"=→"Messgasdruck:":sgl, "aktiver Samplepoint"=→"Entnahmestelle:":i16[], "Amium Zustände"=→"Amium Zustände":T2)
        n89 = Unbundle By Name(w121) -> ("Steuerluft"=w120:bool)
        n90 = Cluster To Array(cluster=w114) -> (array=w113:T7[])
        n91 = for {
          tunnel: w115 -> [w129] mode=indexing
          tunnel: w113 -> [w127] mode=indexing
          tunnel: [w125] -> w112 mode=indexing
          n92 = Unbundle By Name(w129) -> ("Status"=w128:sgl)
          n93 = case shown="0, Standard" w128 {
            tunnel: [1 0] -> w126
            frame 0, Default {
            }
            frame 1..3 {
            }
          }
          n94 = Bundle By Name(cluster=w127, "Regler"=w126) -> (w125:T7)
        }
        n95 = Boolean To (0,1)(Boolean=w120) -> (0, 1=→"Druckluft Störung:":i16)
        n96 = Array To Cluster(array=w112) -> (cluster=w111:T23)
        n97 = local write "Grenzwerte PNS"(w111) -> ()
      }
      event Value Change {
        n98 = event-data() -> ()  [unwired: 7 out]
        n99 = Cluster To Array(cluster="SP") -> (array=w134:bool[])
        n100 = for {
          tunnel: w134 -> [w138] mode=indexing
          shift-right: [w140] -> w133
          shift-left: "" -> [w139]
          i -> [w137]
          n101 = case shown="True" w138 {
            tunnel: [w141 w147] -> w140
            tunnel: w139 -> [w141 w146]
            tunnel: w137 -> [_ w145]
            frame False {
            }
            frame True {
              n102 = Increment(x=w145) -> (x+1=w142:i32)
              n103 = case shown="0..10, Standard" w142 {
                selector: w142 -> [_ _ w150]
                tunnel: ["93" "99" w151] -> w144
                frame 11 {
                }
                frame 12 {
                }
                frame 0..10, Default {
                  n104 = Number To Decimal String(number=w150) -> (decimal integer string=w151:string)  [unwired: 1 in]
                }
              }
              n105 = call <vilib>:"Space Constant.vi"() -> ("String"=w143:string)
              n106 = Concatenate Strings(w146, w143, w144) -> (w147:string)
            }
          }
        }
        n107 = call "Zustände schalten.vi"("Samplepoint setzen"=TRUE, "Samplepoint 2"=w133) -> ()  [unwired: 9 in, 1 out]
      }
    }
  }
